vi "Camera Messenger.vi"(0 "Notifier Name":string, 1 "Binning":u16, 2 "General Camera Actions":T3, 5 "Exposure Time (s)":dbl, 7 "Save Path":path, 9 "No. of Frames":u32, 11 "Camera ROI":T1, 12 "Cooler On?":bool, 13 "Defect Correction On?":bool, 14 "Fan On?":bool) -> (3 "Current Exposure Time (s)":dbl, 4 "Notifier Name Dup":string, 6 "Running?":bool, 8 "Camera ROI":T1, 10 "Current Frame":u32, 15 "Image Ref":T2)   [LabVIEW 2025]
uses:
  Camera Controls/Generic Camera Actions.ctl
  Camera Controls/Generic Camera ROI.ctl
  <vilib>/vision/Image Controls.llb/IMAQ Image.ctl
  Hardware Configuration/Hardware Configuration Controls/Company.ctl
  Hamamatsu/Orca Flash/Orca Flash Controls/Orca Flash ROI.ctl
  Hamamatsu/Orca Flash/Orca Flash Controls/Orca Flash Parameters.ctl
  Hamamatsu/Orca Flash/Orca Flash Controls/Orca Flash Parameter List.ctl
  Hamamatsu/Orca Flash/Orca Flash Controls/Orca Flash Actions.ctl
  IDS/IDS Controls/IDS ROI.ctl
  IDS/IDS Controls/IDS Parameters.ctl
  IDS/IDS Controls/IDS Parameter List.ctl
  IDS/IDS Controls/IDS Actions.ctl
  Photometrics/Prime BSI/PVCam LabView/Prime BSI Type Defs/Prime BSI ROI.ctl
  Photometrics/Prime BSI/PVCam LabView/Prime BSI Type Defs/Prime BSI Parameters.ctl
  Photometrics/Prime BSI/PVCam LabView/Prime BSI Type Defs/Prime BSI Parameter List.ctl
  Photometrics/Prime BSI/PVCam LabView/Prime BSI Type Defs/Prime BSI Actions.ctl
  Camera Controls/Camera IMAQ Key Info.ctl
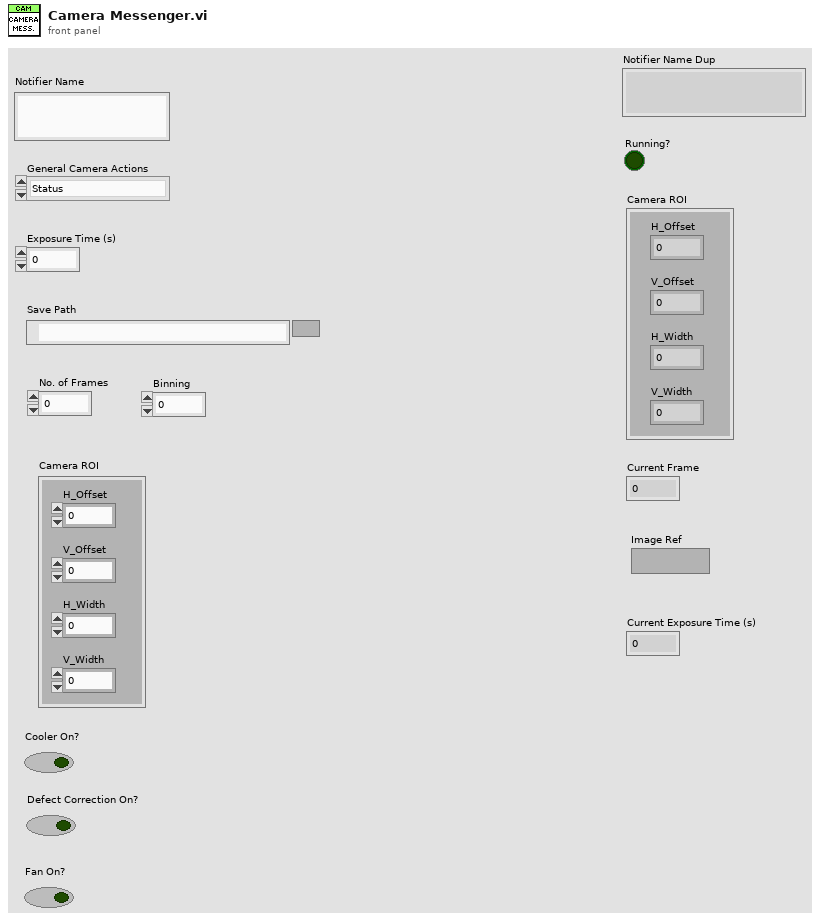
[diagram p1: front panel]
types:
  T1 = typedef "Generic Camera ROI.ctl" = cluster{"H_Offset":u16, "V_Offset":u16, "H_Width":u16, "V_Width":u16}
  T2 = typedef "IMAQ Image.ctl" = refnum<image>
  T3 = typedef "Generic Camera Actions.ctl" = enum16{"Status", "Live Preview", "Capture", "Abort", "Set Exposure Time (s)", "Get Exposure Time (s)", "Record Settings", "Binning", "Set ROI", "Get ROI", "Defect Correction On?", "Cooler On?", "Fan On?", "Quit"}
  T4 = typedef "Company.ctl" = enum16{"AA Opto Electronic", "ASI", "Coherent", "Creset Optics", "CVI", "DAQmx", "Hamamatsu", "IDS", "Mad City Labs", "Marzhauser", "Measurement Computing", "MPB Com", "Olympus", "Photometrics", "PI", "Prior", "Thorlabs"}
  T5 = typedef "Orca Flash Parameters.ctl" = cluster{"Value":dbl, "Parameter":T6}
  T6 = typedef "Orca Flash Parameter List.ctl" = u32
  T7 = typedef "Orca Flash ROI.ctl" = cluster{"H Offset":i32, "V Offset":i32, "H Width":i32, "V Width":i32}
  T8 = typedef "Orca Flash Actions.ctl" = enum16{"Idle", "Preview", "Record", "Record Settings", "Set Param", "Get Param", "Set ROI", "Get ROI", "Trigger Source", "Trigger Type", "Progessive Mode", "Area Mode", "Status", "Quit"}
  T9 = typedef "IDS Parameter List.ctl" = enum16{"Exposure Time (s)", "Binning"}
  T10 = typedef "IDS Parameters.ctl" = cluster{"Parameter":T9, "Value":dbl}
  T11 = typedef "IDS ROI.ctl" = cluster{"H Offset":i32, "V Offset":i32, "H Width":i32, "V Width":i32}
  T12 = typedef "IDS Actions.ctl" = enum16{"Error Check", "Initialize", "Preview", "Record", "Abort", "Record Settings", "Set Parameter", "Get Parameter", "Set ROI", "Get ROI", "Status", "Quit"}
  T13 = typedef "Prime BSI Parameter List.ctl" = enum16{"Exposure Time (s)", "Binning", "Readout Port List", "Available Gain List"}
  T14 = typedef "Prime BSI Parameters.ctl" = cluster{"Parameter":T13, "Value":string[]}
  T15 = typedef "Prime BSI ROI.ctl" = cluster{"H Offset":i32, "V Offset":i32, "H Width":i32, "V Width":i32}
  T16 = typedef "Prime BSI Actions.ctl" = enum16{"Do Nothing", "Preview", "Record", "Abort", "Record Settings", "Set Parameter", "Get Parameter", "Set ROI", "Get ROI", "Status", "Quit"}
  T17 = typedef "Camera IMAQ Key Info.ctl" = cluster{"Frame":u32, "Sensor Height":i32, "Sensor Width":i32, "ROI Height":i32, "ROI Width":i32, "ROI Enable?":bool, "Bit per Pixel":u8}
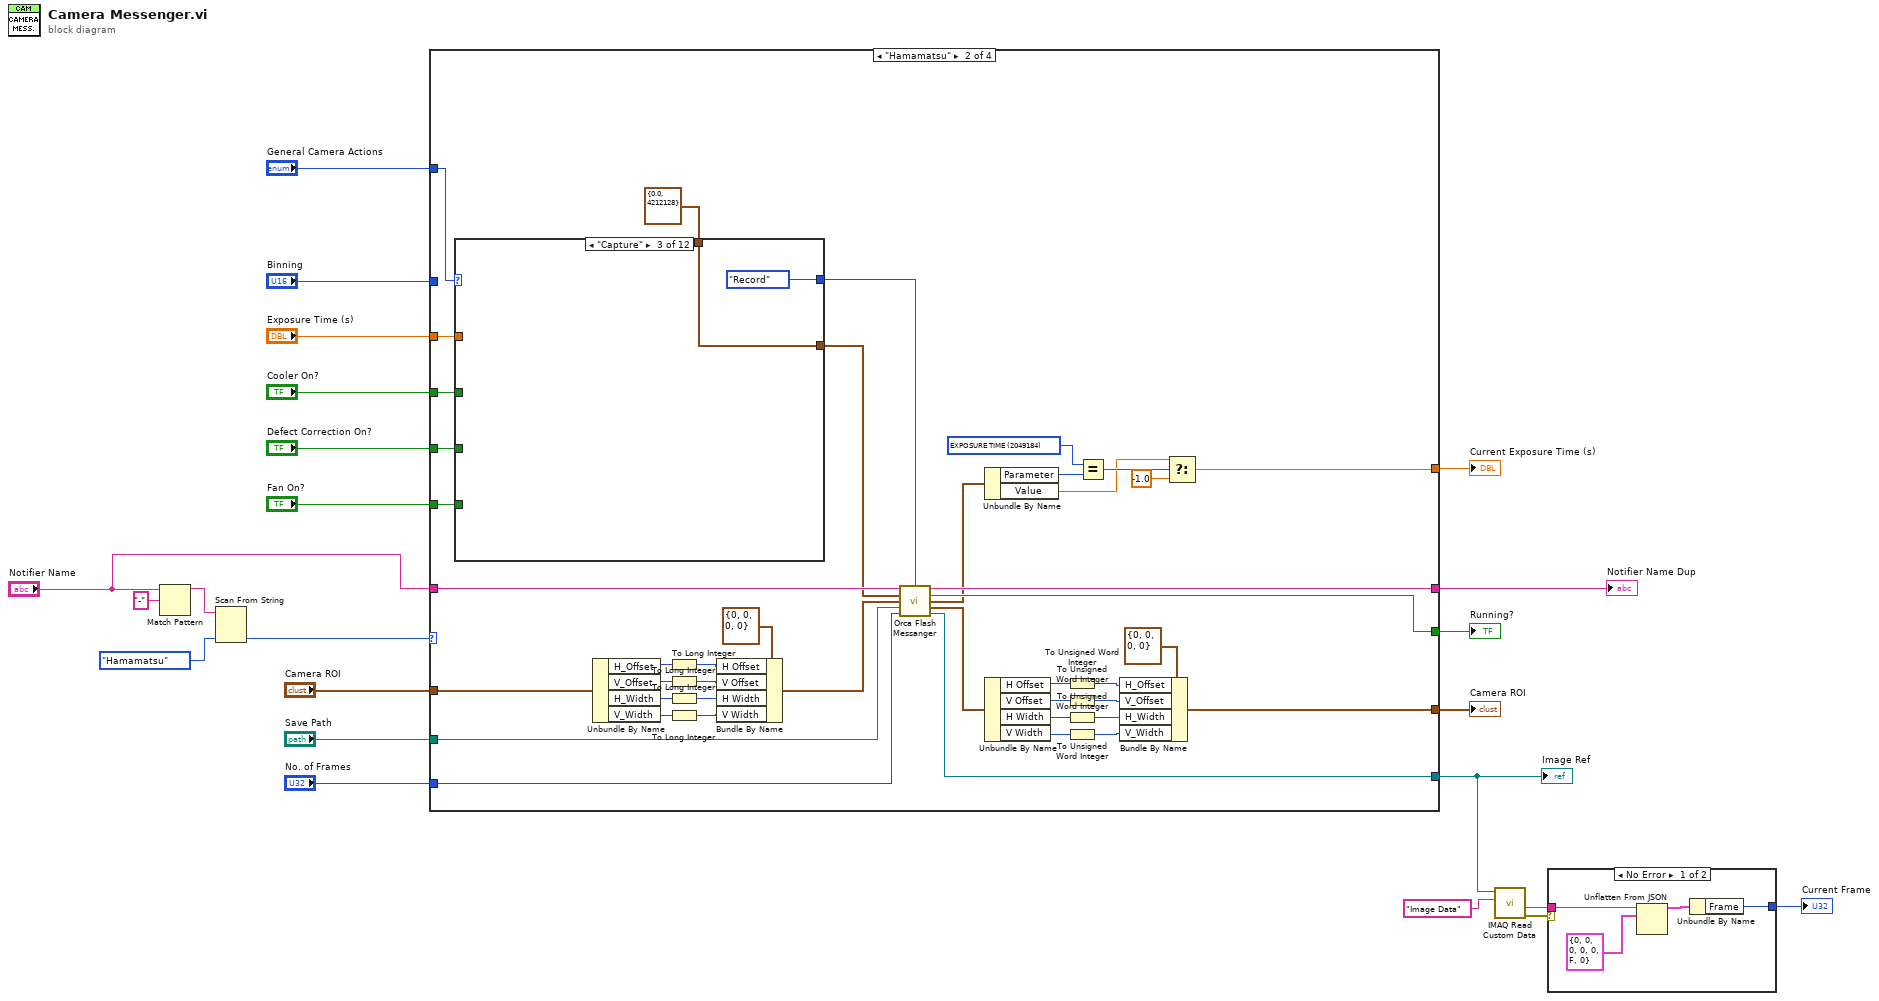
[diagram p0: block diagram]
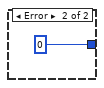
[diagram p2: hidden frame]
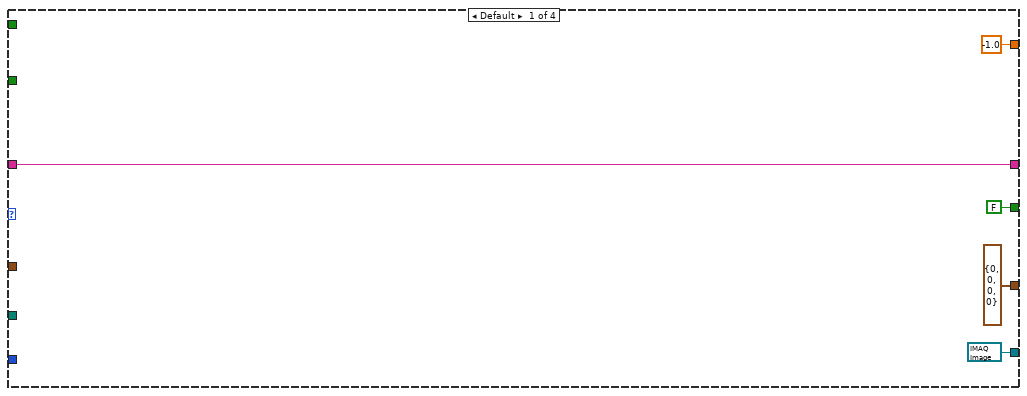
[diagram p3: hidden frame]
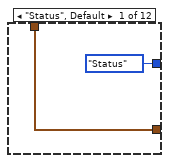
[diagram p4: hidden frame]
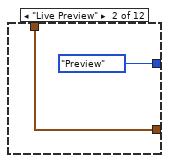
[diagram p5: hidden frame]
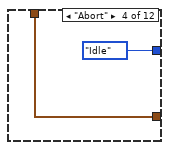
[diagram p6: hidden frame]
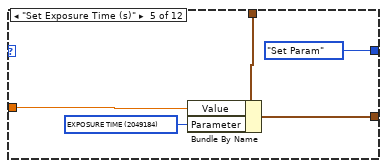
[diagram p7: hidden frame]
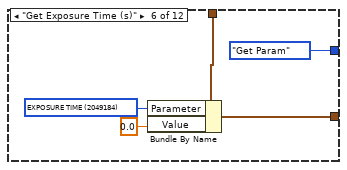
[diagram p8: hidden frame]
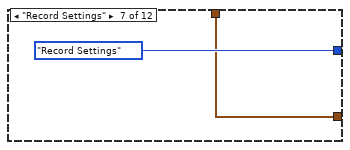
[diagram p9: hidden frame]
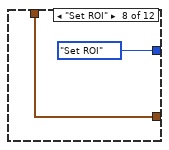
[diagram p10: hidden frame]
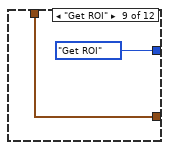
[diagram p11: hidden frame]
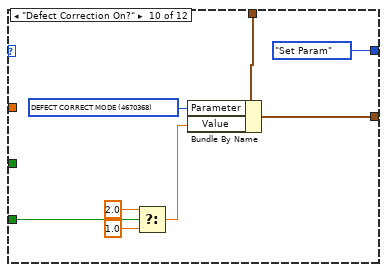
[diagram p12: hidden frame]
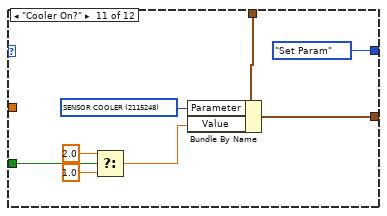
[diagram p13: hidden frame]
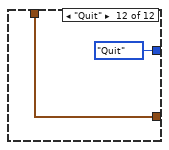
[diagram p14: hidden frame]
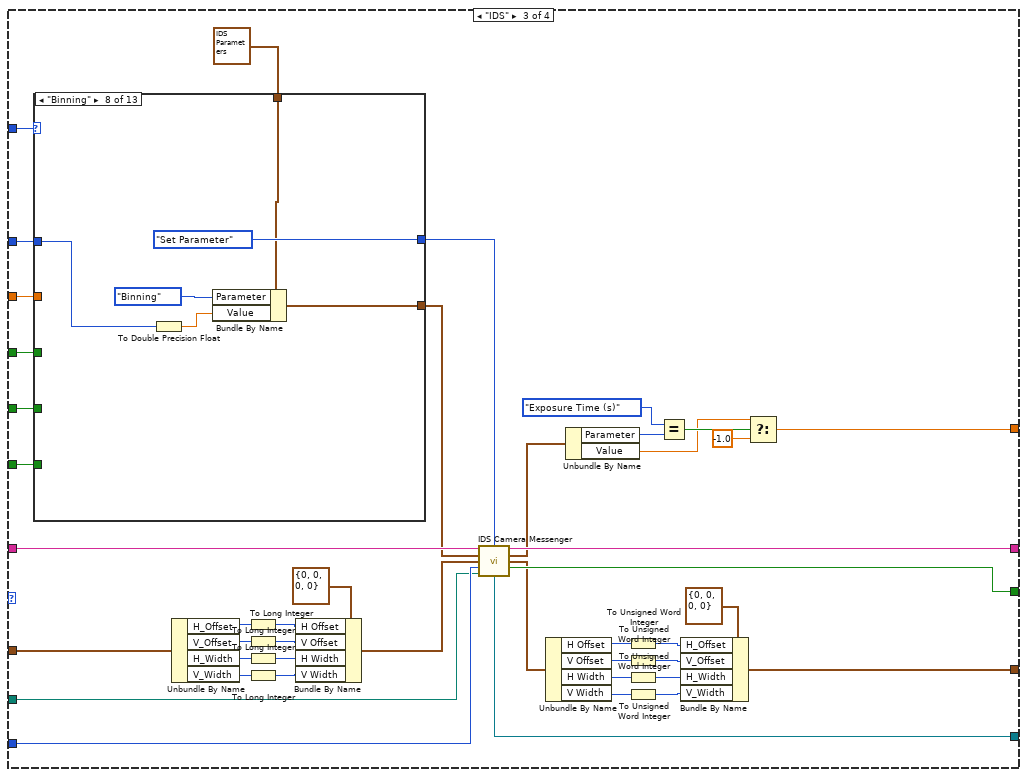
[diagram p15: hidden frame]
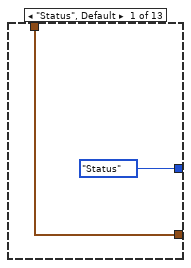
[diagram p16: hidden frame]
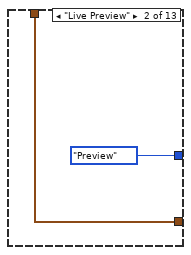
[diagram p17: hidden frame]
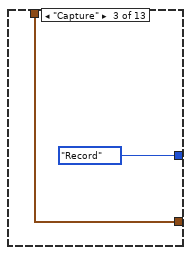
[diagram p18: hidden frame]
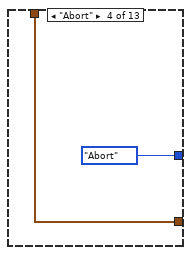
[diagram p19: hidden frame]
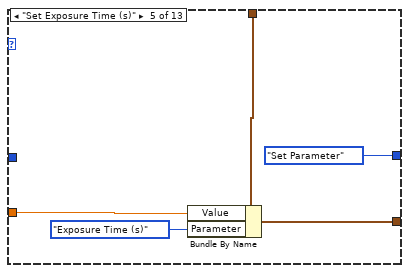
[diagram p20: hidden frame]
diagram:
  n1 = Match Pattern(string="Notifier Name", regular expression="-") -> (before substring=w20:string)  [unwired: 1 in, 3 out]
  n2 = Scan From String(input string=w20, default 1=Company."Hamamatsu" ("Company")) -> (output 1=w21:T4)  [unwired: 3 in, 3 out]
  n3 = case shown="\"Hamamatsu\"" w21 {
    tunnel: "Notifier Name" -> [w28 w71 w157 w240]
    tunnel: "General Camera Actions" -> [_ w56 w142 w235]
    tunnel: "No. of Frames" -> [_ w70 w156 w239]
    tunnel: "Save Path" -> [_ w69 w155 w216]
    tunnel: "Camera ROI" -> [_ w67 w153 w237]
    tunnel: [w28 w57 w143 w236] -> w15
    tunnel: "Exposure Time (s)" -> [_ w51 w138 w231]
    tunnel: "Cooler On?" -> [_ w55 w141 w234]
    tunnel: "Defect Correction On?" -> [_ w54 w140 w233]
    tunnel: "Fan On?" -> [_ w53 w139 w232]
    tunnel: [T2 refnum ("Image Ref") w48 w135 w229] -> w6
    tunnel: [FALSE ("Running?") w47 w134 w228] -> w10
    tunnel: [T1 {"H_Offset"=0, "V_Offset"=0, "H_Width"=0, "V_Width"=0} ("General Camera ROI") w36 w123 w217] -> w9
    tunnel: [-1.0 ("f") w30 w115 w212] -> w2
    tunnel: "Binning" -> [_ _ w114 _]
    frame Default {
    }
    frame "Hamamatsu" {
      w29 = T6 2049184 items=["SENSOR MODE"=4212128, "READOUT SPEED"=4211872, "READOUT DIRECTION"=4211904, "TRIGGER GLOBAL EXPOSURE"=2049680, "TRIGGER DELAY"=1066480, "SYNC READOUT SYSTEM BLANK"=1066528, "SENSOR COOLER"=2115248, "SENSOR COOLER STATUS"=2115280, "EXPOSURE TIME"=2049184, "DEFECT CORRECT MODE"=4670368, "BINNING"=4215968, "INTERNAL LINE SPEED"=4226000, "INTERNAL LINE INTERVAL"=4226016, "IMAGE PIXEL TYPE"=4343296, "NUMBER OF OUTPUT TRIGGER CONNECTOR"=1852320, "OUTPUT TRIGGER SOURCE[0]"=1852576, "OUTPUT TRIGGER SOURCE[1]"=1852832, "OUTPUT TRIGGER SOURCE[2]"=1853088, "OUTPUT TRIGGER POLARITY[0]"=1852592, "OUTPUT TRIGGER POLARITY[1]"=1852848, "OUTPUT TRIGGER POLARITY[2]"=1853104, "OUTPUT TRIGGER ACTIVE[0]"=1852608, "OUTPUT TRIGGER ACTIVE[1]"=1852864, "OUTPUT TRIGGER ACTIVE[2]"=1853120, "OUTPUT TRIGGER DELAY[0]"=1852624, "OUTPUT TRIGGER DELAY[1]"=1852880, "OUTPUT TRIGGER DELAY[2]"=1853136, "OUTPUT TRIGGER PERIOD[0]"=1852640, "OUTPUT TRIGGER PERIOD[1]"=1852896, "OUTPUT TRIGGER PERIOD[2]"=1853152, "OUTPUT TRIGGER KIND[0]"=1852656, "OUTPUT TRIGGER KIND[1]"=1852912, "OUTPUT TRIGGER KIND[2]"=1853168, "OUTPUT TRIGGER PRE HSYNC COUNT"=1852704] ("x")
      n4 = case shown="\"Capture\"" w56 {
        tunnel: w55 -> [_ _ _ _ _ _ _ _ _ _ w109 _]
        tunnel: w54 -> [_ _ _ _ _ _ _ _ _ w100 _ _]
        tunnel: w53 -> [_ _ _ _ _ _ _ _ _ _ _ _]
        tunnel: [Orca_Flash_Actions."Status" ("Camera Actions") Orca_Flash_Actions."Preview" ("Camera Actions") Orca_Flash_Actions."Record" ("Camera Actions") Orca_Flash_Actions."Idle" ("Camera Actions") Orca_Flash_Actions."Set Param" ("Camera Actions") Orca_Flash_Actions."Get Param" ("Camera Actions") Orca_Flash_Actions."Record Settings" ("Camera Actions") Orca_Flash_Actions."Set ROI" ("Camera Actions") Orca_Flash_Actions."Get ROI" ("Camera Actions") Orca_Flash_Actions."Set Param" ("Camera Actions") Orca_Flash_Actions."Set Param" ("Camera Actions") Orca_Flash_Actions."Quit" ("Camera Actions")] -> w52
        tunnel: w51 -> [_ _ _ _ w83 _ _ _ _ _ _ _]
        tunnel: [w73 w74 w76 w78 w82 w88 w90 w92 w94 w101 w105 w113] -> w50
        tunnel: T5 {"Value"=0.0, "Parameter"=4212128} ("sCMOS Parameter") -> [w73 w74 w76 w78 w81 w89 w90 w92 w94 w102 w110 w113]
        frame "Status", Default {
        }
        frame "Live Preview" {
        }
        frame "Capture" {
        }
        frame "Abort" {
        }
        frame "Set Exposure Time (s)" {
          w80 = T6 2049184 items=["SENSOR MODE"=4212128, "READOUT SPEED"=4211872, "READOUT DIRECTION"=4211904, "TRIGGER GLOBAL EXPOSURE"=2049680, "TRIGGER DELAY"=1066480, "SYNC READOUT SYSTEM BLANK"=1066528, "SENSOR COOLER"=2115248, "SENSOR COOLER STATUS"=2115280, "EXPOSURE TIME"=2049184, "DEFECT CORRECT MODE"=4670368, "BINNING"=4215968, "INTERNAL LINE SPEED"=4226000, "INTERNAL LINE INTERVAL"=4226016, "IMAGE PIXEL TYPE"=4343296, "NUMBER OF OUTPUT TRIGGER CONNECTOR"=1852320, "OUTPUT TRIGGER SOURCE[0]"=1852576, "OUTPUT TRIGGER SOURCE[1]"=1852832, "OUTPUT TRIGGER SOURCE[2]"=1853088, "OUTPUT TRIGGER POLARITY[0]"=1852592, "OUTPUT TRIGGER POLARITY[1]"=1852848, "OUTPUT TRIGGER POLARITY[2]"=1853104, "OUTPUT TRIGGER ACTIVE[0]"=1852608, "OUTPUT TRIGGER ACTIVE[1]"=1852864, "OUTPUT TRIGGER ACTIVE[2]"=1853120, "OUTPUT TRIGGER DELAY[0]"=1852624, "OUTPUT TRIGGER DELAY[1]"=1852880, "OUTPUT TRIGGER DELAY[2]"=1853136, "OUTPUT TRIGGER PERIOD[0]"=1852640, "OUTPUT TRIGGER PERIOD[1]"=1852896, "OUTPUT TRIGGER PERIOD[2]"=1853152, "OUTPUT TRIGGER KIND[0]"=1852656, "OUTPUT TRIGGER KIND[1]"=1852912, "OUTPUT TRIGGER KIND[2]"=1853168, "OUTPUT TRIGGER PRE HSYNC COUNT"=1852704, "OPM Trigger"=0] ("Parameter")
          n5 = Bundle By Name(cluster=w81, "Value"=w83, "Parameter"=w80) -> (w82:T5)
        }
        frame "Get Exposure Time (s)" {
          w85 = T6 2049184 items=["SENSOR MODE"=4212128, "READOUT SPEED"=4211872, "READOUT DIRECTION"=4211904, "TRIGGER GLOBAL EXPOSURE"=2049680, "TRIGGER DELAY"=1066480, "SYNC READOUT SYSTEM BLANK"=1066528, "SENSOR COOLER"=2115248, "SENSOR COOLER STATUS"=2115280, "EXPOSURE TIME"=2049184, "DEFECT CORRECT MODE"=4670368, "BINNING"=4215968, "INTERNAL LINE SPEED"=4226000, "INTERNAL LINE INTERVAL"=4226016, "IMAGE PIXEL TYPE"=4343296, "NUMBER OF OUTPUT TRIGGER CONNECTOR"=1852320, "OUTPUT TRIGGER SOURCE[0]"=1852576, "OUTPUT TRIGGER SOURCE[1]"=1852832, "OUTPUT TRIGGER SOURCE[2]"=1853088, "OUTPUT TRIGGER POLARITY[0]"=1852592, "OUTPUT TRIGGER POLARITY[1]"=1852848, "OUTPUT TRIGGER POLARITY[2]"=1853104, "OUTPUT TRIGGER ACTIVE[0]"=1852608, "OUTPUT TRIGGER ACTIVE[1]"=1852864, "OUTPUT TRIGGER ACTIVE[2]"=1853120, "OUTPUT TRIGGER DELAY[0]"=1852624, "OUTPUT TRIGGER DELAY[1]"=1852880, "OUTPUT TRIGGER DELAY[2]"=1853136, "OUTPUT TRIGGER PERIOD[0]"=1852640, "OUTPUT TRIGGER PERIOD[1]"=1852896, "OUTPUT TRIGGER PERIOD[2]"=1853152, "OUTPUT TRIGGER KIND[0]"=1852656, "OUTPUT TRIGGER KIND[1]"=1852912, "OUTPUT TRIGGER KIND[2]"=1853168, "OUTPUT TRIGGER PRE HSYNC COUNT"=1852704, "OPM Trigger"=0] ("Parameter")
          n6 = Bundle By Name(cluster=w89, "Parameter"=w85, "Value"=0.0) -> (w88:T5)
        }
        frame "Record Settings" {
        }
        frame "Set ROI" {
        }
        frame "Get ROI" {
        }
        frame "Defect Correction On?" {
          w96 = T6 4670368 items=["SENSOR MODE"=4212128, "READOUT SPEED"=4211872, "READOUT DIRECTION"=4211904, "TRIGGER GLOBAL EXPOSURE"=2049680, "TRIGGER DELAY"=1066480, "SYNC READOUT SYSTEM BLANK"=1066528, "SENSOR COOLER"=2115248, "SENSOR COOLER STATUS"=2115280, "EXPOSURE TIME"=2049184, "DEFECT CORRECT MODE"=4670368, "BINNING"=4215968, "INTERNAL LINE SPEED"=4226000, "INTERNAL LINE INTERVAL"=4226016, "IMAGE PIXEL TYPE"=4343296, "NUMBER OF OUTPUT TRIGGER CONNECTOR"=1852320, "OUTPUT TRIGGER SOURCE[0]"=1852576, "OUTPUT TRIGGER SOURCE[1]"=1852832, "OUTPUT TRIGGER SOURCE[2]"=1853088, "OUTPUT TRIGGER POLARITY[0]"=1852592, "OUTPUT TRIGGER POLARITY[1]"=1852848, "OUTPUT TRIGGER POLARITY[2]"=1853104, "OUTPUT TRIGGER ACTIVE[0]"=1852608, "OUTPUT TRIGGER ACTIVE[1]"=1852864, "OUTPUT TRIGGER ACTIVE[2]"=1853120, "OUTPUT TRIGGER DELAY[0]"=1852624, "OUTPUT TRIGGER DELAY[1]"=1852880, "OUTPUT TRIGGER DELAY[2]"=1853136, "OUTPUT TRIGGER PERIOD[0]"=1852640, "OUTPUT TRIGGER PERIOD[1]"=1852896, "OUTPUT TRIGGER PERIOD[2]"=1853152, "OUTPUT TRIGGER KIND[0]"=1852656, "OUTPUT TRIGGER KIND[1]"=1852912, "OUTPUT TRIGGER KIND[2]"=1853168, "OUTPUT TRIGGER PRE HSYNC COUNT"=1852704, "OPM Trigger"=0] ("Parameter")
          n7 = Select(t=2.0, s=w100, f=1.0) -> (s? t:f=w97:dbl)
          n8 = Bundle By Name(cluster=w102, "Parameter"=w96, "Value"=w97) -> (w101:T5)
        }
        frame "Cooler On?" {
          w104 = T6 2115248 items=["SENSOR MODE"=4212128, "READOUT SPEED"=4211872, "READOUT DIRECTION"=4211904, "TRIGGER GLOBAL EXPOSURE"=2049680, "TRIGGER DELAY"=1066480, "SYNC READOUT SYSTEM BLANK"=1066528, "SENSOR COOLER"=2115248, "SENSOR COOLER STATUS"=2115280, "EXPOSURE TIME"=2049184, "DEFECT CORRECT MODE"=4670368, "BINNING"=4215968, "INTERNAL LINE SPEED"=4226000, "INTERNAL LINE INTERVAL"=4226016, "IMAGE PIXEL TYPE"=4343296, "NUMBER OF OUTPUT TRIGGER CONNECTOR"=1852320, "OUTPUT TRIGGER SOURCE[0]"=1852576, "OUTPUT TRIGGER SOURCE[1]"=1852832, "OUTPUT TRIGGER SOURCE[2]"=1853088, "OUTPUT TRIGGER POLARITY[0]"=1852592, "OUTPUT TRIGGER POLARITY[1]"=1852848, "OUTPUT TRIGGER POLARITY[2]"=1853104, "OUTPUT TRIGGER ACTIVE[0]"=1852608, "OUTPUT TRIGGER ACTIVE[1]"=1852864, "OUTPUT TRIGGER ACTIVE[2]"=1853120, "OUTPUT TRIGGER DELAY[0]"=1852624, "OUTPUT TRIGGER DELAY[1]"=1852880, "OUTPUT TRIGGER DELAY[2]"=1853136, "OUTPUT TRIGGER PERIOD[0]"=1852640, "OUTPUT TRIGGER PERIOD[1]"=1852896, "OUTPUT TRIGGER PERIOD[2]"=1853152, "OUTPUT TRIGGER KIND[0]"=1852656, "OUTPUT TRIGGER KIND[1]"=1852912, "OUTPUT TRIGGER KIND[2]"=1853168, "OUTPUT TRIGGER PRE HSYNC COUNT"=1852704, "OPM Trigger"=0] ("Parameter")
          n9 = Select(t=2.0, s=w109, f=1.0) -> (s? t:f=w106:dbl)
          n10 = Bundle By Name(cluster=w110, "Parameter"=w104, "Value"=w106) -> (w105:T5)
        }
        frame "Quit" {
        }
      }
      n11 = Unbundle By Name(w67) -> ("H_Offset"=w63:u16, "V_Offset"=w64:u16, "H_Width"=w65:u16, "V_Width"=w66:u16)
      n12 = To Long Integer(number=w63) -> (32bit integer=w62:i32)
      n13 = To Long Integer(number=w64) -> (32bit integer=w61:i32)
      n14 = To Long Integer(number=w65) -> (32bit integer=w60:i32)
      n15 = To Long Integer(number=w66) -> (32bit integer=w59:i32)
      n16 = Bundle By Name(cluster=T7 {"H Offset"=0, "V Offset"=0, "H Width"=0, "V Width"=0} ("sCMOS ROI"), "H Offset"=w62, "V Offset"=w61, "H Width"=w60, "V Width"=w59) -> (w58:T7)
      n17 = call "Orca Flash Messanger.vi"("Notifier Name"=w71, "Camera Actions"=w52, "sCMOS Parameter"=w50, "sCMOS ROI"=w58, "Path"=w69, "# of frames"=w70) -> ("Notifier Name Dup"=w57:string, "Running?"=w47:bool, "sCMOS Parameter"=w31:T5, "sCMOS ROI"=w45:T7, "Image Ref"=w48:T2)  [unwired: 5 in]
      n18 = Unbundle By Name(w31) -> ("Parameter"=w35:T6, "Value"=w33:dbl)
      n19 = Unbundle By Name(w45) -> ("H Offset"=w44:i32, "V Offset"=w43:i32, "H Width"=w42:i32, "V Width"=w41:i32)
      n20 = To Unsigned Word Integer(number=w44) -> (unsigned 16bit integer=w40:u16)
      n21 = To Unsigned Word Integer(number=w43) -> (unsigned 16bit integer=w39:u16)
      n22 = To Unsigned Word Integer(number=w42) -> (unsigned 16bit integer=w38:u16)
      n23 = To Unsigned Word Integer(number=w41) -> (unsigned 16bit integer=w37:u16)
      n24 = Equal?(x=w29, y=w35) -> (x = y?=w34:bool)
      n25 = Bundle By Name(cluster=T1 {"H_Offset"=0, "V_Offset"=0, "H_Width"=0, "V_Width"=0} ("General Camera ROI"), "H_Offset"=w40, "V_Offset"=w39, "H_Width"=w38, "V_Width"=w37) -> (w36:T1)
      n26 = Select(t=w33, s=w34, f=-1.0) -> (s? t:f=w30:dbl)
    }
    frame "IDS" {
      n27 = case shown="\"Binning\"" w142 {
        tunnel: w141 -> [_ _ _ _ _ _ _ _ _ _ _ _ _]
        tunnel: w140 -> [_ _ _ _ _ _ _ _ _ _ _ _ _]
        tunnel: w139 -> [_ _ _ _ _ _ _ _ _ _ _ _ _]
        tunnel: [IDS_Actions."Status" ("IDS Actions") IDS_Actions."Preview" ("IDS Actions") IDS_Actions."Record" ("IDS Actions") IDS_Actions."Abort" ("IDS Actions") IDS_Actions."Set Parameter" ("IDS Actions") IDS_Actions."Get Parameter" ("IDS Actions") IDS_Actions."Record Settings" ("IDS Actions") IDS_Actions."Set Parameter" ("IDS Actions") IDS_Actions."Set ROI" ("IDS Actions") IDS_Actions."Get ROI" ("IDS Actions") IDS_Actions."Status" ("IDS Actions") IDS_Actions."Status" ("IDS Actions") IDS_Actions."Quit" ("IDS Actions")] -> w122
        tunnel: w138 -> [_ _ _ _ w170 _ _ _ _ _ _ _ _]
        tunnel: [w159 w161 w163 w165 w169 w171 w177 w181 w185 w187 w189 w191 w193] -> w137
        tunnel: T10 {"Parameter"=enum."Exposure Time (s)", "Value"=4212128.0} ("IDS Parameter") -> [w159 w161 w163 w165 w168 w174 w177 w182 w185 w187 w189 w191 w193]
        tunnel: w114 -> [_ _ _ _ _ _ _ w178 _ _ _ _ _]
        frame "Status", Default {
        }
        frame "Live Preview" {
        }
        frame "Capture" {
        }
        frame "Abort" {
        }
        frame "Set Exposure Time (s)" {
          n28 = Bundle By Name(cluster=w168, "Value"=w170, "Parameter"=IDS_Parameter_List."Exposure Time (s)") -> (w169:T10)
        }
        frame "Get Exposure Time (s)" {
          n29 = Bundle By Name(cluster=w174, "Parameter"=IDS_Parameter_List."Exposure Time (s)", "Value"=0.0) -> (w171:T10)
        }
        frame "Record Settings" {
        }
        frame "Binning" {
          n30 = To Double Precision Float(number=w178) -> (double precision float=w179:dbl)
          n31 = Bundle By Name(cluster=w182, "Parameter"=IDS_Parameter_List."Binning", "Value"=w179) -> (w181:T10)
        }
        frame "Set ROI" {
        }
        frame "Get ROI" {
        }
        frame "Defect Correction On?" {
        }
        frame "Cooler On?" {
        }
        frame "Quit" {
        }
      }
      n32 = Unbundle By Name(w153) -> ("H_Offset"=w149:u16, "V_Offset"=w150:u16, "H_Width"=w151:u16, "V_Width"=w152:u16)
      n33 = To Long Integer(number=w149) -> (32bit integer=w148:i32)
      n34 = To Long Integer(number=w150) -> (32bit integer=w147:i32)
      n35 = To Long Integer(number=w151) -> (32bit integer=w146:i32)
      n36 = To Long Integer(number=w152) -> (32bit integer=w145:i32)
      n37 = Bundle By Name(cluster=T11 {"H Offset"=0, "V Offset"=0, "H Width"=0, "V Width"=0} ("sCMOS ROI"), "H Offset"=w148, "V Offset"=w147, "H Width"=w146, "V Width"=w145) -> (w144:T11)
      n38 = call "IDS Camera Messenger.vi"("Notifier Name"=w157, "IDS Actions"=w122, "IDS Parameter"=w137, "ROI Setup"=w144, "# of Frames"=w156, "File Save Path"=w155) -> ("Notifier Name (Dup)"=w143:string, "IDS Parameter"=w121:T10, "IDS ROI"=w132:T11, "Running?"=w134:bool, "Image Ref"=w135:T2)  [unwired: 4 in, 1 out]
      n39 = Unbundle By Name(w132) -> ("H Offset"=w131:i32, "V Offset"=w130:i32, "H Width"=w129:i32, "V Width"=w128:i32)
      n40 = Unbundle By Name(w121) -> ("Parameter"=w120:T9, "Value"=w117:dbl)
      n41 = To Unsigned Word Integer(number=w131) -> (unsigned 16bit integer=w127:u16)
      n42 = To Unsigned Word Integer(number=w130) -> (unsigned 16bit integer=w126:u16)
      n43 = To Unsigned Word Integer(number=w129) -> (unsigned 16bit integer=w125:u16)
      n44 = To Unsigned Word Integer(number=w128) -> (unsigned 16bit integer=w124:u16)
      n45 = Equal?(x=IDS_Parameter_List."Exposure Time (s)", y=w120) -> (x = y?=w118:bool)
      n46 = Bundle By Name(cluster=T1 {"H_Offset"=0, "V_Offset"=0, "H_Width"=0, "V_Width"=0} ("General Camera ROI"), "H_Offset"=w127, "V_Offset"=w126, "H_Width"=w125, "V_Width"=w124) -> (w123:T1)
      n47 = Select(t=w117, s=w118, f=-1.0) -> (s? t:f=w115:dbl)
    }
    frame "Photometrics" {
      w194 = -1.0 ("f")
      n48 = case shown="\"Set Exposure Time (s)\"" w235 {
        tunnel: w234 -> [_ _ _ _ _ _ _ _ _ _ _ _]
        tunnel: w233 -> [_ _ _ _ _ _ _ _ _ _ _ _]
        tunnel: w232 -> [_ _ _ _ _ _ _ _ _ _ _ _]
        tunnel: [Prime_BSI_Actions."Status" ("PVCam Actions") Prime_BSI_Actions."Preview" ("PVCam Actions") Prime_BSI_Actions."Record" ("PVCam Actions") Prime_BSI_Actions."Abort" ("PVCam Actions") Prime_BSI_Actions."Set Parameter" ("PVCam Actions") Prime_BSI_Actions."Get Parameter" ("PVCam Actions") Prime_BSI_Actions."Record Settings" ("PVCam Actions") Prime_BSI_Actions."Set ROI" ("PVCam Actions") Prime_BSI_Actions."Get ROI" ("PVCam Actions") Prime_BSI_Actions."Status" ("PVCam Actions") Prime_BSI_Actions."Status" ("PVCam Actions") Prime_BSI_Actions."Quit" ("PVCam Actions")] -> w210
        tunnel: w231 -> [_ _ _ _ w251 _ _ _ _ _ _ _]
        tunnel: [w242 w244 w246 w248 w256 w260 w264 w266 w268 w270 w272 w274] -> w209
        tunnel: T14 {"Parameter"=enum."Exposure Time (s)", "Value"=[]} ("PVCam Parameter") -> [w242 w244 w246 w248 w255 w261 w264 w266 w268 w270 w272 w274]
        frame "Status", Default {
        }
        frame "Live Preview" {
        }
        frame "Capture" {
        }
        frame "Abort" {
        }
        frame "Set Exposure Time (s)" {
          n49 = Format Value(format string="%f", value (0)=w251) -> (output string=w250:string)  [unwired: 1 in]
          n50 = Build Array(w250) -> (w249:string[])
          n51 = Bundle By Name(cluster=w255, "Value"=w249, "Parameter"=Prime_BSI_Parameter_List."Exposure Time (s)") -> (w256:T14)
        }
        frame "Get Exposure Time (s)" {
          n52 = Build Array("") -> (w257:string[])
          n53 = Bundle By Name(cluster=w261, "Parameter"=Prime_BSI_Parameter_List."Exposure Time (s)", "Value"=w257) -> (w260:T14)
        }
        frame "Record Settings" {
        }
        frame "Set ROI" {
        }
        frame "Get ROI" {
        }
        frame "Defect Correction On?" {
        }
        frame "Cooler On?" {
        }
        frame "Quit" {
        }
      }
      n54 = Unbundle By Name(w237) -> ("V_Offset"=w208:u16, "V_Width"=w206:u16, "H_Offset"=w205:u16, "H_Width"=w204:u16)
      n55 = To Long Integer(number=w208) -> (32bit integer=w207:i32)
      n56 = To Long Integer(number=w206) -> (32bit integer=w203:i32)
      n57 = To Long Integer(number=w205) -> (32bit integer=w202:i32)
      n58 = To Long Integer(number=w204) -> (32bit integer=w201:i32)
      n59 = Bundle By Name(cluster=T15 {"H Offset"=0, "V Offset"=0, "H Width"=0, "V Width"=0} ("sCMOS ROI"), "V Offset"=w207, "V Width"=w203, "H Offset"=w202, "H Width"=w201) -> (w211:T15)
      n60 = call "Prime BSI Camera Messenger.vi"("Notifier Name"=w240, "Prime Actions"=w210, "Prime Parameter"=w209, "ROI Setup"=w211, "# of Frames"=w239, "File Save Path"=w216) -> ("Notifier Name (Dup)"=w236:string, "Prime Parameter"=w213:T14, "Prime ROI"=w226:T15, "Running?"=w228:bool, "Image Ref"=w229:T2)  [unwired: 4 in, 1 out]
      n61 = Unbundle By Name(w213) -> ("Parameter"=w215:T13, "Value"=w199:string[])
      n62 = Unbundle By Name(w226) -> ("H Offset"=w225:i32, "V Offset"=w224:i32, "H Width"=w223:i32, "V Width"=w222:i32)
      n63 = To Unsigned Word Integer(number=w225) -> (unsigned 16bit integer=w221:u16)
      n64 = To Unsigned Word Integer(number=w224) -> (unsigned 16bit integer=w220:u16)
      n65 = To Unsigned Word Integer(number=w223) -> (unsigned 16bit integer=w219:u16)
      n66 = To Unsigned Word Integer(number=w222) -> (unsigned 16bit integer=w218:u16)
      n67 = Equal?(x=Prime_BSI_Parameter_List."Exposure Time (s)", y=w215) -> (x = y?=w214:bool)
      n68 = Index Array(array=w199, index=0) -> (element=w196:string)
      n69 = Bundle By Name(cluster=T1 {"H_Offset"=0, "V_Offset"=0, "H_Width"=0, "V_Width"=0} ("General Camera ROI"), "H_Offset"=w221, "V_Offset"=w220, "H_Width"=w219, "V_Width"=w218) -> (w217:T1)
      n70 = Scan Value(string=w196, format string="%f", default (0 dbl)=w194) -> (value=w195:dbl)  [unwired: 1 out]
      n71 = Select(t=w195, s=w214, f=w194) -> (s? t:f=w212:dbl)
    }
  }
  "Notifier Name Dup" <- w15
  "Image Ref" <- w6
  "Running?" <- w10
  "Camera ROI" <- w9
  "Current Exposure Time (s)" <- w2
  n72 = call "IMAQ Read Custom Data"("Key"="Image Data", "Image"=w6) -> ("error out"=w5:errorcluster, "Custom Data Out"=w7:string)  [unwired: 7 in, 1 out]
  n73 = case shown="No Error" w5 {
    tunnel: w7 -> [w278 _]
    tunnel: [w275 u32 0 ("Frame")] -> w4
    frame No Error {
      n74 = Unflatten From JSON(JSON string=w278, type and defaults=T17 {"Frame"=0, "Sensor Height"=0, "Sensor Width"=0, "ROI Height"=0, "ROI Width"=0, "ROI Enable?"=FALSE, "Bit per Pixel"=0} ("Camera IMAQ Key Info")) -> (value=w276:T17)  [unwired: 5 in, 1 out]
      n75 = Unbundle By Name(w276) -> ("Frame"=w275:u32)
    }
    frame Error {
    }
  }
  "Current Frame" <- w4
